vi "Reset node.vi"() -> ()   [LabVIEW 2016]
uses:
  <vilib>/CANopenLib/CANOPEN.llb/CANopen Interface Close.vi
panel:
  out "Used Node ID":u8 min=1 max=127 step=1
  out "error out":errorcluster
  in  "Motor":u8(ring) items=["Right", "Left"]
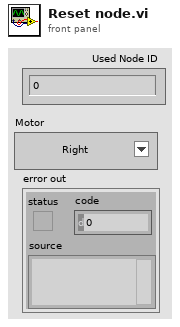
[diagram p1: front panel]
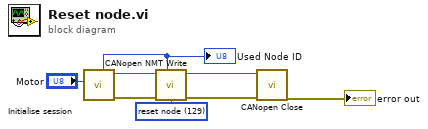
[diagram p0: block diagram]
diagram:
  w7 = u16 129 items=["start remote node"=1, "stop remote node"=2, "enter pre-operational"=128, "reset node"=129, "reset communication"=130] ("command")
  n1 = call "Initialise session.vi"("Motor"="Motor") -> ("error out"=w6:errorcluster, "interface object out"=w5:refnum<k20>, "Used Node ID"=w4:u8)  [unwired: 8 in]
  "Used Node ID" <- w4
  n2 = call <vilib>:"CANopen NMT Write.vi"("node-ID (0)"=w4, "error in (no error)"=w6, "command"=w7, "interface object in"=w5) -> ("error out"=w3:errorcluster, "interface object out"=w2:refnum<k20>)  [unwired: 6 in]
  n3 = call-poly <vilib>:"CANopen Close.vi"("error in (no error)"=w3, "interface object in"=w2) -> ("error out"=→"error out":errorcluster)  [unwired: 9 in]
